vi "prueba sonido.vi"() -> ()   [LabVIEW 2010]
uses:
  <vilib>/sound2/lvsound2.llb/Sound Data Format.ctl
  <vilib>/sound2/lvsound2.llb/Sampling Mode.ctl
  <vilib>/sound2/lvsound2.llb/Sound Output Write (DBL Single).vi
panel:
  out "Ultimo":dbl
  out "Inicial":dbl
  out "1/x":sgl
  out "x*y":dbl
  out "#samples":u32
  in  "frequency":dbl=10.0 format="%0.2p"
  out "Generated Sound":waveform(dbl)(graph)={"t0"=timestamp(1.2471655328798186 s since 1904-01-01), "dt"=2.2675736961451248e-05, "Y"=[]}
  in  "sound format":T1={"sample rate (S/s)"=22050.0, "number of channels"=2, "bits per sample"=16}
  in  "tiempo (ms)":u32=100
  in  "stop 2":bool
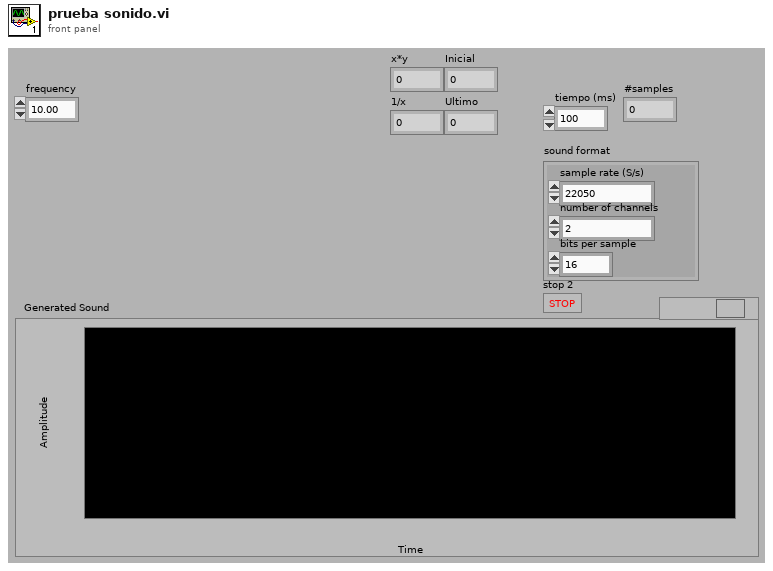
[diagram p1: front panel]
types:
  T1 = typedef "Sound Data Format.ctl" = cluster{"sample rate (S/s)":dbl, "number of channels":i32, "bits per sample":i32}
  T2 = typedef "Sampling Mode.ctl" = i32
  T3 = typedef "Sound Output Task ID.ctl" = u32
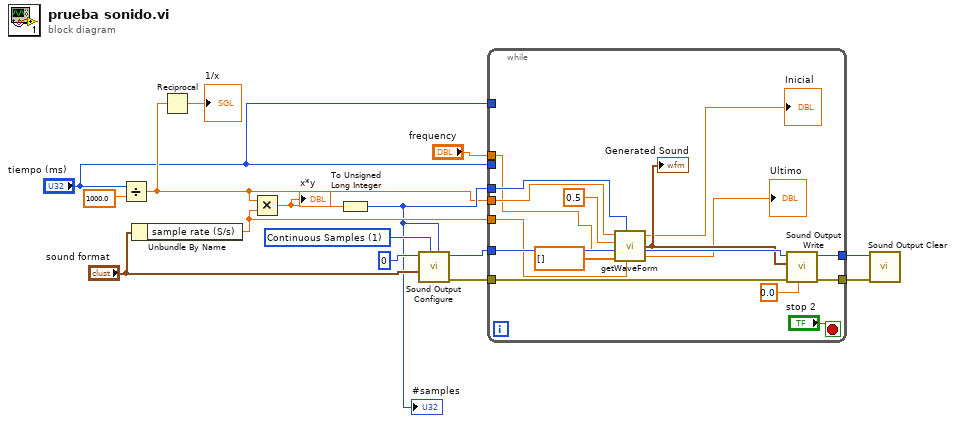
[diagram p0: block diagram]
diagram:
  w15 = T2 1 items=["Finite Samples", "Continuous Samples"] ("sample mode")
  n1 = Divide(x="tiempo (ms)", y=sgl 1000.0) -> (x/y=w3:sgl)
  n2 = Unbundle By Name("sound format") -> ("sample rate (S/s)"=w6:dbl)
  n3 = Reciprocal(x=w3) -> (1/x=→"1/x":sgl)
  n4 = Multiply(x=w3, y=w6) -> (x*y=w4:dbl)
  "x*y" <- w4
  n5 = To Unsigned Long Integer(number=w4) -> (unsigned 32bit integer=w5:u32)
  "#samples" <- w5
  n6 = call <vilib>:"Sound Output Configure.vi"("number of samples/ch"=w5, "sample mode"=w15, "sound format"="sound format", "device ID"=u32 0) -> ("error out"=w12:errorcluster, "task ID"=w13:T3)  [unwired: 6 in]
  n7 = while {
    tunnel: w13 -> [w30]
    tunnel: w12 -> [w29]
    tunnel: [w28] -> w11
    tunnel: [w27] -> w10
    tunnel: "tiempo (ms)" -> [_]
    tunnel: "frequency" -> [w19]
    tunnel: w6 -> [w24]
    tunnel: w5 -> [w23]
    tunnel: w3 -> [w21]
    tunnel: "tiempo (ms)" -> [_]
    stop <- "stop 2" stop-if-true
    n8 = call "getWaveForm.vi"("tiempo (s)"=w21, "#samples"=w23, "Amplitud"=0.5, "frecuencia"=w19, "Fs (S/s)"=w24, "df"=dbl[] []) -> ("Inicial"=→"Inicial":dbl, "Waveform"=w25:waveform(dbl), "Ultimo"=→"Ultimo":dbl)
    "Generated Sound" <- w25
    n9 = call-poly <vilib>:"Sound Output Write.vi"("timeout (sec)"=0.0, "error in (no error)"=w29, "data"=w25, "task ID"=w30) -> ("error out"=w27:errorcluster, "task ID out"=w28:T3)  [unwired: 6 in]
  }
  n10 = call <vilib>:"Sound Output Clear.vi"("error in (no error)"=w10, "task ID"=w11) -> ()  [unwired: 9 in, 1 out]
